vi "Send.vi"(8 "error in (no error)":errorcluster, 10 "Tx String":string, 11 "Message Transport Queue in":refnum<class "Message Transport Queue.lvclass">) -> (0 "error out":errorcluster)   [LabVIEW 2016, in "Parrot Msg.lvclass"]
doc: "--\nCopyright © 2017 Composed SystemsI All rights reserved.\n\nAuthor: Jon McBee <jon.mcbee@composed.io>\n\nThis library is provided \"AS IS\" ,WITHOUT WARRANTIES OR\nCONDITIONS OF ANY KIND, either express or implied.\n\nComposed Systems -- composed.io\n\nStream 0.0.1.1\nJon McBee - Composed Systems\nCopyright (c) 2017, Composed Systems"
uses:
  <userlib>/Composed Systems/Stream/Sandbox/Async Actor Test/Parrot Msg/Parrot Msg.lvclass
  <userlib>/Composed Systems/Stream/Mediator/Classes/Message Transport Queue/Message Transport Queue.lvclass
  D:/Repos/Stream/software/Mediator/Classes/Message Interface/Message Interface.lvclass
  <userlib>/Composed Systems/Stream/Sandbox/Async Actor Test/Parrot Msg/Parrot Msg.lvclass/Parrot Msg.ctl
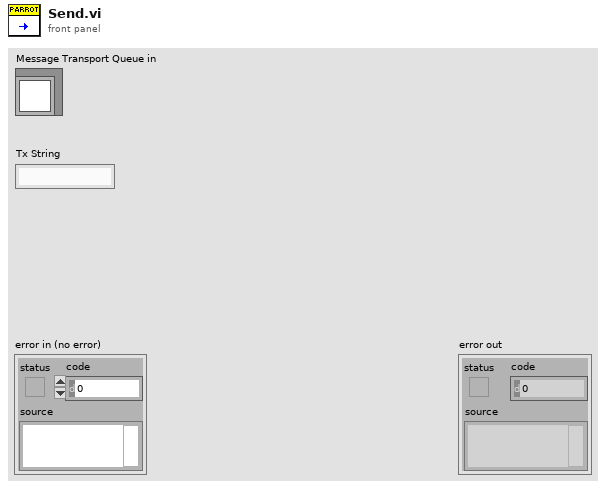
[diagram p1: front panel]
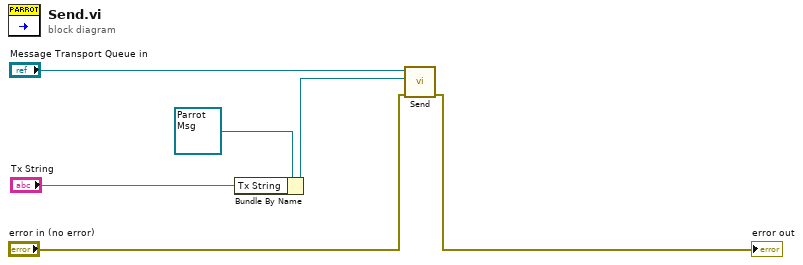
[diagram p0: block diagram]
diagram:
  n1 = Bundle By Name(cluster=refnum<class "Parrot Msg.lvclass"> refnum ("Parrot Msg in"), "Tx String"="Tx String") -> (w4:refnum<class "Parrot Msg.lvclass">)
  n2 = call-dynamic "Send.vi"("error in (no error)"="error in (no error)", "Message"=w4, "Message Transport Queue in"="Message Transport Queue in") -> ("error out"=→"error out":errorcluster)  [unwired: 6 in, 2 out]
